vi "Trav_Cluster_to_Row.vi"(4 "Traverse line in":T1 {"Carrier_2 Q (l/min)" format="%#.2f"; "Row Duration (mins)" format="%#.1f"; "Row No" min=0; "Trace Gas Concentration (%)" min=0.0 format="%#_4f"; "Carrier_1 Q (l/min)" format="%#.4f"; "Start X" format="%#.2f"; "Start Y" format="%#.2f"; "Start Z" format="%#.2f"; "End X" format="%#.2f"; "End Y" format="%#.2f"; "End Z" format="%#.2f"; "Tunnel Speed" format="%#.2f"; "Averaging time (mins)" min=0.0 format="%#.2f"}, 6 "Row Number":i32, 7 "Channel names":string[](array[string])) -> (0 "Traverse line Out":T1 {"Carrier_2 Q (l/min)" format="%#.2f"; "Row Duration (mins)" format="%#.1f"; "Row No" min=0; "Trace Gas Concentration (%)" min=0.0 format="%#_4f"; "Carrier_1 Q (l/min)" format="%#.4f"; "Start X" format="%#.2f"; "Start Y" format="%#.2f"; "Start Z" format="%#.2f"; "End X" format="%#.2f"; "End Y" format="%#.2f"; "End Z" format="%#.2f"; "Tunnel Speed" format="%#.2f"; "Averaging time (mins)" min=0.0 format="%#.2f"}, 1 "Channel Values Out":string[](array[string]))   [LabVIEW 2020]
uses:
  Traverse_cluster.ctl
  Spacing.ctl
  Controls/Multi_run_mode.ctl
  Globals/Trav_pos_global.vi
  Globals/Meas_global.vi
panel:
  # "X           Y          Z"
  # "Start"
  # "End"
  # "X           Y          Z"
  # "Start"
  # "End"
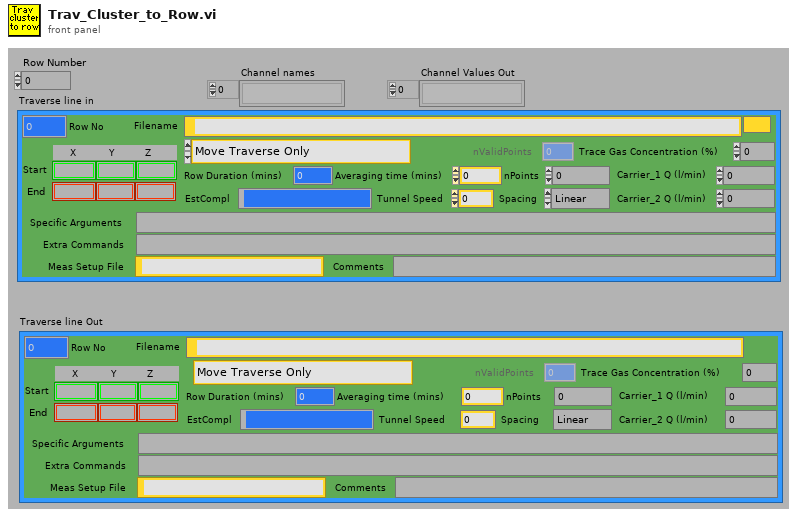
[diagram p1: front panel]
types:
  T1 = typedef "Traverse_cluster.ctl" = cluster{"Start X":sgl, "Start Y":sgl, "Start Z":sgl, "End X":sgl, "End Y":sgl, "End Z":sgl, "nPoints":i32, "Spacing":T2, "Filename":path, "Tunnel Speed":dbl, "Averaging time (mins)":dbl, "Extra Commands":string, "Carrier_1 Q (l/min)":dbl, "Carrier_2 Q (l/min)":dbl, "Trace Gas Concentration (%)":dbl, "Specific Arguments":string, "Comments":string, "Row No":i32, "Row Type Selector":T3, "EstCompl":string, "Row Duration (mins)":dbl, "nValidPoints":i32, "Meas Setup File":string}
  T2 = typedef "Spacing.ctl" = enum16{"Linear", "Log", "Gauss", "Specified", "N/A"}
  T3 = typedef "Multi_run_mode.ctl" = enum16{"Move Traverse Only", "Set Tunnel Speed Only", "Set Source Only", "Set Measurement Conditions", "Single Measurement", "Vertical Profile", "Lateral Profile", "Longitudinal Profile", "Multi-Axis Profile", "Explore Volume", "Auto Calibrate", "Meas Fast FID Bkgnd", "Check Beam Power", "Scanning Valve Measurement", "Run VI Named:", "Set ADAM Ch", "Wait (minutes)", "Send Message", "Synchronize With:", "Fall Back to this Row", "Turn Off Row Repeating", "Traverse 3D Volume", "Blank Row", "Jump to Fall Back Row"}
  T4 = enum16{"All Channel Names", "Valid Channel Names"}
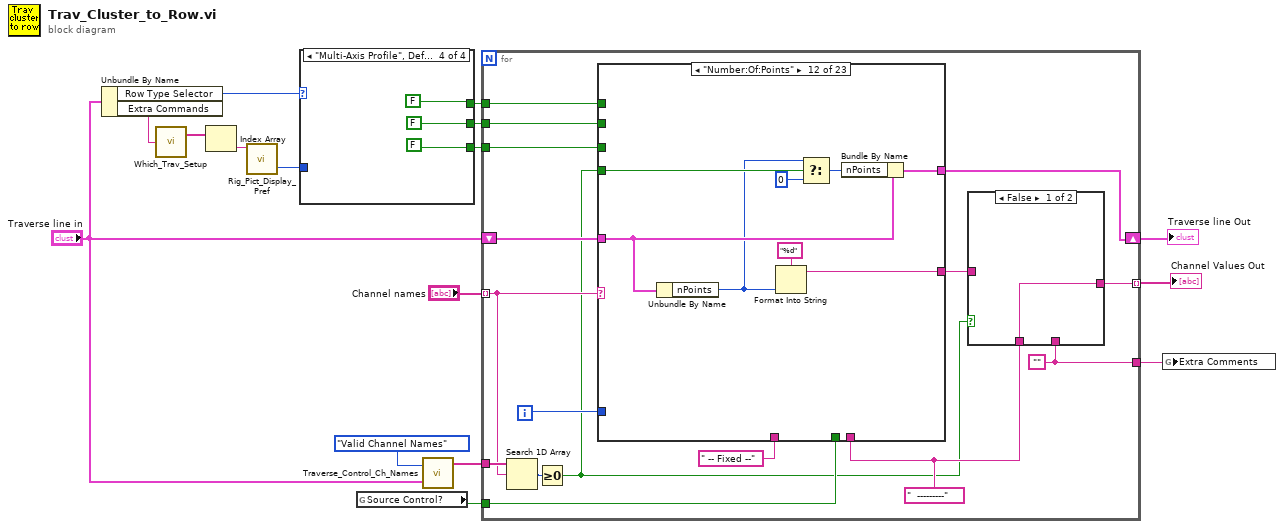
[diagram p0: block diagram]
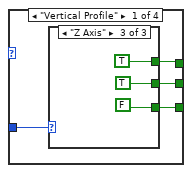
[diagram p2: hidden frame]
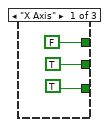
[diagram p3: hidden frame]
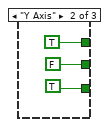
[diagram p4: hidden frame]
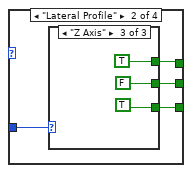
[diagram p5: hidden frame]
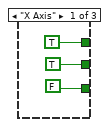
[diagram p6: hidden frame]
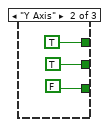
[diagram p7: hidden frame]
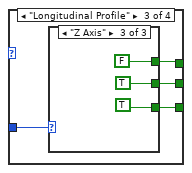
[diagram p8: hidden frame]
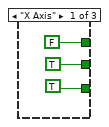
[diagram p9: hidden frame]
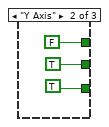
[diagram p10: hidden frame]
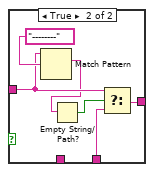
[diagram p11: hidden frame]
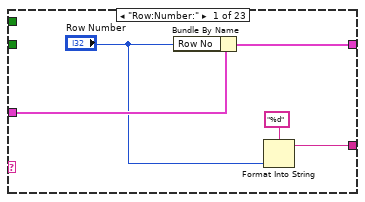
[diagram p12: hidden frame]
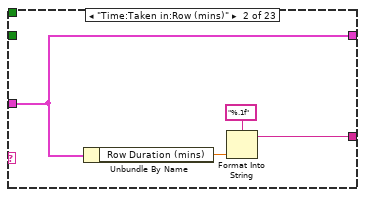
[diagram p13: hidden frame]
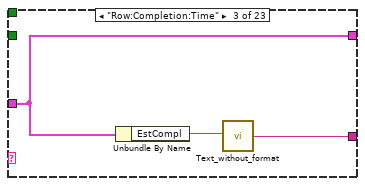
[diagram p14: hidden frame]
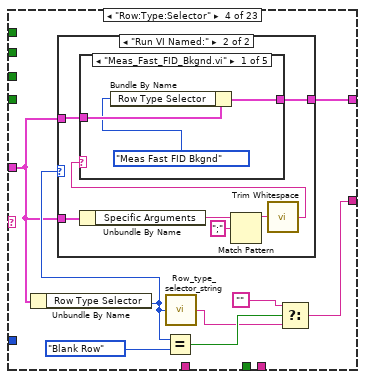
[diagram p15: hidden frame]
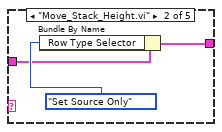
[diagram p17: hidden frame]
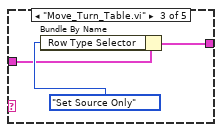
[diagram p18: hidden frame]
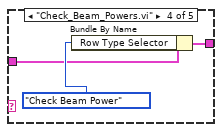
[diagram p19: hidden frame]
diagram:
  n1 = Unbundle By Name("Traverse line in") -> ("Row Type Selector"=w8:T3, "Extra Commands"=w3:string)
  n2 = call "Which_Trav_Setup.vi"("Extra Command String"=w3) -> ("Traverse Setups"=w2:string[])  [unwired: 2 out]
  n3 = Index Array(array=w2) -> (element=w1:string)  [unwired: 1 in]
  n4 = call "Rig_Pict_Display_Pref.vi"("Traverse Name"=w1) -> ("Which Axis is vertical?"=w9:enum16{"X Axis", "Y Axis", "Z Axis"})  [unwired: 7 out]
  n5 = case shown="\"Multi-Axis Profile\", Default" w8 {
    tunnel: [w20 w33 w46 FALSE] -> w7
    tunnel: [w19 w32 w45 FALSE] -> w6
    tunnel: [w18 w31 w44 FALSE] -> w5
    tunnel: w9 -> [w17 w30 w43 _]
    frame "Vertical Profile" {
      n6 = case shown="\"Z Axis\"" w17 {
        tunnel: [FALSE TRUE TRUE] -> w20
        tunnel: [TRUE FALSE TRUE] -> w19
        tunnel: [TRUE TRUE FALSE] -> w18
        frame "X Axis" {
        }
        frame "Y Axis" {
        }
        frame "Z Axis" {
        }
      }
    }
    frame "Lateral Profile" {
      n7 = case shown="\"Z Axis\"" w30 {
        tunnel: [TRUE TRUE TRUE] -> w33
        tunnel: [TRUE TRUE FALSE] -> w32
        tunnel: [FALSE FALSE TRUE] -> w31
        frame "X Axis" {
        }
        frame "Y Axis" {
        }
        frame "Z Axis" {
        }
      }
    }
    frame "Longitudinal Profile" {
      n8 = case shown="\"Z Axis\"" w43 {
        tunnel: [FALSE FALSE FALSE] -> w46
        tunnel: [TRUE TRUE TRUE] -> w45
        tunnel: [TRUE TRUE TRUE] -> w44
        frame "X Axis" {
        }
        frame "Y Axis" {
        }
        frame "Z Axis" {
        }
      }
    }
    frame "Multi-Axis Profile", Default {
    }
  }
  n9 = global read "Trav_pos_global.vi" "Source Control?"() -> (w13:bool)
  n10 = call "Traverse_Control_Ch_Names.vi"("Traverse line"="Traverse line in", "Mode"=T4."Valid Channel Names") -> ("Channel names"=w14:string[])
  n11 = for {
    tunnel: "Channel names" -> [w72] mode=indexing
    tunnel: [w68] -> w16 mode=indexing
    shift-right: [w64] -> w10
    shift-left: "Traverse line in" -> [w74]
    tunnel: w14 -> [w73]
    tunnel: w13 -> [w70]
    tunnel: [w65] -> w11
    tunnel: w7 -> [w62]
    tunnel: w6 -> [w60]
    tunnel: w5 -> [w59]
    i -> [w69]
    w65 = ""
    w66 = "  ---------" ("f")
    n12 = Search 1D Array(1D array=w73, element=w72) -> (index of element=w71:i32)  [unwired: 1 out]
    n13 = Greater Or Equal To 0?(x=w71) -> (x >= 0?=w63:bool)
    n14 = case shown="\"Number:Of:Points\"" w72 {
      selector: w72 -> [_ _ _ _ _ _ _ _ _ _ _ _ _ _ _ _ _ _ _ _ _ _ w300]
      tunnel: w74 -> [w83 w87 w93 w94 w128 w137 w144 w153 w164 w175 w186 w192 w199 w214 w226 w228 w245 w255 w266 w277 w288 w298 w301]
      tunnel: [w85 w89 w91 w98 w127 w135 w143 w151 w160 w170 w181 w194 w200 w216 w221 w229 w237 w252 w263 w274 w281 w291 ""] -> w67
      tunnel: [w84 w87 w93 w95 w129 w136 w145 w152 w163 w174 w185 w193 w197 w215 w225 w235 w244 w256 w267 w278 w289 w299 w301] -> w64
      tunnel: w70 -> [_ _ _ _ _ _ _ _ _ _ _ _ _ _ _ _ _ w254 w265 w275 _ _ _]
      tunnel: w69 -> [_ _ _ _ _ _ _ _ _ _ _ _ _ _ _ _ _ _ _ _ _ _ _]
      tunnel: w66 -> [_ _ _ _ _ _ _ _ _ _ _ _ _ _ w223 w227 w239 w251 w262 w273 w282 w292 _]
      tunnel: w63 -> [_ _ _ _ w125 w133 w139 w148 w158 w168 w179 w190 w196 w212 w224 w231 w240 w249 w260 w271 w284 w294 _]
      tunnel: w62 -> [_ _ _ _ _ _ _ _ w162 _ _ _ _ _ _ _ _ _ _ _ _ _ _]
      tunnel: " -- Fixed --" ("t") -> [_ _ _ _ _ _ _ _ w159 w173 w183 _ _ _ _ _ _ _ _ _ _ _ _]
      tunnel: w60 -> [_ _ _ _ _ _ _ _ _ w172 _ _ _ _ _ _ _ _ _ _ _ _ _]
      tunnel: w59 -> [_ _ _ _ _ _ _ _ _ _ w184 _ _ _ _ _ _ _ _ _ _ _ _]
      frame "Row:Number:" {
        n15 = Bundle By Name(cluster=w83, "Row No"="Row Number") -> (w84:T1)
        n16 = Format Into String(format string="%d", "Row Number") -> (resulting string=w85:string)  [unwired: 2 in, 1 out]
      }
      frame "Time:Taken in:Row (mins)" {
        n17 = Unbundle By Name(w87) -> ("Row Duration (mins)"=w88:dbl)
        n18 = Format Into String(format string="%.1f", w88) -> (resulting string=w89:string)  [unwired: 2 in, 1 out]
      }
      frame "Row:Completion:Time" {
        n19 = Unbundle By Name(w93) -> ("EstCompl"=w92:string)
        n20 = call "Text_without_format.vi"("Input string"=w92) -> ("Output string"=w91:string)
      }
      frame "Row:Type:Selector" {
        n21 = Unbundle By Name(w94) -> ("Row Type Selector"=w96:T3)
        n22 = case shown="\"Run VI Named:\"" w96 {
          tunnel: w94 -> [_ w109]
          tunnel: [w102 w108] -> w95
          tunnel: w94 -> [w102 w107]
          frame "Move Traverse Only", Default {
          }
          frame "Run VI Named:" {
            n23 = Unbundle By Name(w109) -> ("Specific Arguments"=w105:string)
            n24 = Match Pattern(string=w105, regular expression=";") -> (before substring=w104:string)  [unwired: 4 out]
            n25 = call <vilib>:"Trim Whitespace.vi"("string"=w104) -> ("trimmed string"=w103:string)  [unwired: 1 in]
            n26 = case shown="\"Meas_Fast_FID_Bkgnd.vi\"" w103 {
              tunnel: [w110 w113 w116 w119 w122] -> w108
              tunnel: w107 -> [w112 w114 w117 w120 w122]
              frame "Meas_Fast_FID_Bkgnd.vi" {
                n27 = Bundle By Name(cluster=w112, "Row Type Selector"=Multi_run_mode."Meas Fast FID Bkgnd" ("Mode")) -> (w110:T1)
              }
              frame "Move_Stack_Height.vi" {
                n28 = Bundle By Name(cluster=w114, "Row Type Selector"=Multi_run_mode."Set Source Only" ("Mode")) -> (w113:T1)
              }
              frame "Move_Turn_Table.vi" {
                n29 = Bundle By Name(cluster=w117, "Row Type Selector"=Multi_run_mode."Set Source Only" ("Mode")) -> (w116:T1)
              }
              frame "Check_Beam_Powers.vi" {
                n30 = Bundle By Name(cluster=w120, "Row Type Selector"=Multi_run_mode."Check Beam Power" ("Mode")) -> (w119:T1)
              }
              frame "No Match", Default {
              }
            }
          }
        }
        n31 = Equal?(x=w96, y=Multi_run_mode."Blank Row" ("Mode")) -> (x = y?=w100:bool)
        n32 = call "Row_type_selector_string.vi"("Mode"=w96) -> ("Output string"=w99:string)
        n33 = Select(t="", s=w100, f=w99) -> (s? t:f=w98:string)
      }
      frame "Tunnel:Speed:(m/s)" {
        n34 = Unbundle By Name(w128) -> ("Tunnel Speed"=w124:dbl)
        n35 = Format Into String(format string="%f", w124) -> (resulting string=w127:string)  [unwired: 2 in, 1 out]
        n36 = Select(t=w124, s=w125, f=nan) -> (s? t:f=w123:dbl)
        n37 = Bundle By Name(cluster=w128, "Tunnel Speed"=w123) -> (w129:T1)
      }
      frame "Start at:X:(mm)" {
        n38 = Unbundle By Name(w137) -> ("Start X"=w131:sgl)
        n39 = Select(t=w131, s=w133, f=nan) -> (s? t:f=w132:dbl)
        n40 = Format Into String(format string="%.3f", w131) -> (resulting string=w135:string)  [unwired: 2 in, 1 out]
        n41 = Bundle By Name(cluster=w137, "Start X"=w132) -> (w136:T1)
      }
      frame "Start at:Y:(mm)" {
        n42 = Unbundle By Name(w144) -> ("Start Y"=w140:sgl)
        n43 = Select(t=w140, s=w139, f=nan) -> (s? t:f=w141:dbl)
        n44 = Format Into String(format string="%.3f", w140) -> (resulting string=w143:string)  [unwired: 2 in, 1 out]
        n45 = Bundle By Name(cluster=w144, "Start Y"=w141) -> (w145:T1)
      }
      frame "Start at:Z:(mm)" {
        n46 = Unbundle By Name(w153) -> ("Start Z"=w149:sgl)
        n47 = Select(t=w149, s=w148, f=nan) -> (s? t:f=w147:dbl)
        n48 = Format Into String(format string="%.3f", w149) -> (resulting string=w151:string)  [unwired: 2 in, 1 out]
        n49 = Bundle By Name(cluster=w153, "Start Z"=w147) -> (w152:T1)
      }
      frame "End at:X:(mm)" {
        n50 = Unbundle By Name(w164) -> ("End X"=w155:sgl)
        n51 = Format Into String(format string="%.3f", w155) -> (resulting string=w161:string)  [unwired: 2 in, 1 out]
        n52 = Select(t=w155, s=w158, f=nan) -> (s? t:f=w156:dbl)
        n53 = Bundle By Name(cluster=w164, "End X"=w156) -> (w163:T1)
        n54 = Select(t=w159, s=w162, f=w161) -> (s? t:f=w160:string)
      }
      frame "End at:Y:(mm)" {
        n55 = Unbundle By Name(w175) -> ("End Y"=w167:sgl)
        n56 = Format Into String(format string="%.3f", w167) -> (resulting string=w171:string)  [unwired: 2 in, 1 out]
        n57 = Select(t=w167, s=w168, f=nan) -> (s? t:f=w166:dbl)
        n58 = Bundle By Name(cluster=w175, "End Y"=w166) -> (w174:T1)
        n59 = Select(t=w173, s=w172, f=w171) -> (s? t:f=w170:string)
      }
      frame "End at:Z:(mm)" {
        n60 = Unbundle By Name(w186) -> ("End Z"=w178:sgl)
        n61 = Format Into String(format string="%.3f", w178) -> (resulting string=w182:string)  [unwired: 2 in, 1 out]
        n62 = Select(t=w178, s=w179, f=nan) -> (s? t:f=w177:dbl)
        n63 = Select(t=w183, s=w184, f=w182) -> (s? t:f=w181:string)
        n64 = Bundle By Name(cluster=w186, "End Z"=w177) -> (w185:T1)
      }
      frame "Number:Of:Points" {
        n65 = Unbundle By Name(w192) -> ("nPoints"=w188:i32)
        n66 = Format Into String(format string="%d", w188) -> (resulting string=w194:string)  [unwired: 2 in, 1 out]
        n67 = Select(t=w188, s=w190, f=0 ("t")) -> (s? t:f=w191:i32)
        n68 = Bundle By Name(cluster=w192, "nPoints"=w191) -> (w193:T1)
      }
      frame "Point:Spacing:Method" {
        n69 = Unbundle By Name(w199) -> ("Spacing"=w198:T2)
        n70 = case shown="False" w196 {
          tunnel: w199 -> [w203 w204]
          tunnel: [w201 w204] -> w197
          frame False {
            n71 = Bundle By Name(cluster=w203, "Spacing"=Spacing."N/A") -> (w201:T1)
          }
          frame True {
          }
        }
        n72 = case shown="\"N/A\"" w198 {
          tunnel: ["Linear" "Log" "Gauss" "Specified" "N/A"] -> w200
          frame "Linear" {
          }
          frame "Log" {
          }
          frame "Gauss" {
          }
          frame "Specified" {
          }
          frame "N/A" {
          }
        }
      }
      frame "Averaging:Time:(mins)" {
        n73 = Unbundle By Name(w214) -> ("Averaging time (mins)"=w210:dbl)
        n74 = Select(t=w210, s=w212, f=nan) -> (s? t:f=w211:dbl)
        n75 = Bundle By Name(cluster=w214, "Averaging time (mins)"=w211) -> (w215:T1)
        n76 = Format Into String(format string="%.2f", w210) -> (resulting string=w216:string)  [unwired: 2 in, 1 out]
      }
      frame "Filename:HD:Users" {
        n77 = Unbundle By Name(w226) -> ("Filename"=w219:path)
        n78 = Strip Path(path=w219) -> (name=w218:string)  [unwired: 1 out]
        n79 = call "Text_without_format.vi"("Input string"=w218) -> ("Output string"=w221:string)
        n80 = Select(t=w221, s=w224, f=w223) -> (s? t:f=w222:string)
        n81 = String To Path(string=w222) -> (path=w220:path)
        n82 = Bundle By Name(cluster=w226, "Filename"=w220) -> (w225:T1)
      }
      frame "Specific:Arguments:String" {
        n83 = Unbundle By Name(w228) -> ("Specific Arguments"=w236:string)
        n84 = call "Text_without_format.vi"("Input string"=w236) -> ("Output string"=w232:string)
        n85 = Not Equal?(x=w232, y=w227) -> (x != y?=w234:bool)
        n86 = Select(t=w232, s=w234, f="") -> (s? t:f=w229:string)
        n87 = Select(t=w229, s=w231, f=w227) -> (s? t:f=w230:string)
        n88 = Bundle By Name(cluster=w228, "Specific Arguments"=w230) -> (w235:T1)
      }
      frame "Extra:Commands:String" {
        n89 = Unbundle By Name(w245) -> ("Extra Commands"=w246:string)
        n90 = call "Text_without_format.vi"("Input string"=w246) -> ("Output string"=w241:string)
        n91 = Not Equal?(x=w241, y=w239) -> (x != y?=w243:bool)
        n92 = Select(t=w241, s=w243, f="") -> (s? t:f=w237:string)
        n93 = Select(t=w237, s=w240, f=w239) -> (s? t:f=w238:string)
        n94 = Bundle By Name(cluster=w245, "Extra Commands"=w238) -> (w244:T1)
      }
      frame "Carrier_1:Q:(l/min)" {
        n95 = Unbundle By Name(w255) -> ("Carrier_1 Q (l/min)"=w248:dbl)
        n96 = Select(t=w248, s=w249, f=nan) -> (s? t:f=w247:dbl)
        n97 = Format Into String(format string="%.4f", w248) -> (resulting string=w253:string)  [unwired: 2 in, 1 out]
        n98 = Bundle By Name(cluster=w255, "Carrier_1 Q (l/min)"=w247) -> (w256:T1)
        n99 = Select(t=w253, s=w254, f=w251) -> (s? t:f=w252:string)
      }
      frame "Carrier_2:Q:(l/min)" {
        n100 = Unbundle By Name(w266) -> ("Carrier_2 Q (l/min)"=w259:dbl)
        n101 = Select(t=w259, s=w260, f=nan) -> (s? t:f=w258:dbl)
        n102 = Format Into String(format string="%.3f", w259) -> (resulting string=w264:string)  [unwired: 2 in, 1 out]
        n103 = Bundle By Name(cluster=w266, "Carrier_2 Q (l/min)"=w258) -> (w267:T1)
        n104 = Select(t=w264, s=w265, f=w262) -> (s? t:f=w263:string)
      }
      frame "Trace Gas:Concentration:(%)" {
        n105 = Unbundle By Name(w277) -> ("Trace Gas Concentration (%)"=w270:dbl)
        n106 = Select(t=w270, s=w271, f=nan) -> (s? t:f=w269:dbl)
        n107 = Bundle By Name(cluster=w277, "Trace Gas Concentration (%)"=w269) -> (w278:T1)
        n108 = Format Into String(format string="%.3f", w270) -> (resulting string=w276:string)  [unwired: 2 in, 1 out]
        n109 = Select(t=w276, s=w275, f=w273) -> (s? t:f=w274:string)
      }
      frame "Comments::" {
        n110 = Unbundle By Name(w288) -> ("Comments"=w280:string)
        n111 = call "Text_without_format.vi"("Input string"=w280) -> ("Output string"=w285:string)
        n112 = Not Equal?(x=w285, y=w282) -> (x != y?=w287:bool)
        n113 = Select(t=w285, s=w287, f="") -> (s? t:f=w281:string)
        n114 = Select(t=w281, s=w284, f=w282) -> (s? t:f=w283:string)
        n115 = Bundle By Name(cluster=w288, "Comments"=w283) -> (w289:T1)
      }
      frame "Measurement:Setup:File" {
        n116 = Unbundle By Name(w298) -> ("Meas Setup File"=w290:string)
        n117 = call "Text_without_format.vi"("Input string"=w290) -> ("Output string"=w295:string)
        n118 = Not Equal?(x=w295, y=w292) -> (x != y?=w297:bool)
        n119 = Select(t=w295, s=w297, f="") -> (s? t:f=w291:string)
        n120 = Select(t=w291, s=w294, f=w292) -> (s? t:f=w293:string)
        n121 = Bundle By Name(cluster=w298, "Meas Setup File"=w293) -> (w299:T1)
      }
      frame "No match", Default {
        n122 = call "Was_string_matched.vi"("Variable name"=w300) -> ()  [unwired: 2 in]
      }
    }
    n123 = case shown="False" w63 {
      tunnel: [w75 w80] -> w68
      tunnel: w67 -> [_ w78]
      tunnel: w66 -> [w75 _]
      tunnel: w65 -> [_ w81]
      frame False {
      }
      frame True {
        n124 = Match Pattern(string=w78, regular expression="--------" ("f")) -> (match substring=w77:string)  [unwired: 4 out]
        n125 = Empty String/Path?(string/path=w77) -> (empty?=w76:bool)
        n126 = Select(t=w78, s=w76, f=w81) -> (s? t:f=w80:string)
      }
    }
  }
  "Channel Values Out" <- w16
  "Traverse line Out" <- w10
  n127 = global write "Meas_global.vi" "Extra Comments"(w11) -> ()
